vi "Get Compatible Interfaces.vi"(8 "error in (no error)":errorcluster, 10 "Interface Filter":T1[](array[typedef]), 11 "fpga resources":T3[](array[typedef]) {"fpga cd" format="%.0x"}) -> (0 "error out":errorcluster, 2 "Compatible Interface Names":string[](array[string]), 3 "fpga resources out":T3[](array[typedef]) {"fpga cd" format="%.0x"})   [LabVIEW 2016, in "FPGA RM System Definition API.lvlib"]
uses:
  FPGA RM System Definition API.lvlib
  Types/resources.ctl
  <vilib>/NI Veristand/Custom Device API/Custom Device Item Ref.ctl
  Types/fpga resource.ctl
  Types/Channel Type.ctl
  Shared/Requested Resource.ctl
  Shared/FPGA RM Shared API.lvlib
  <vilib>/NI VeriStand/Custom Device API/Custom Device API.lvlib
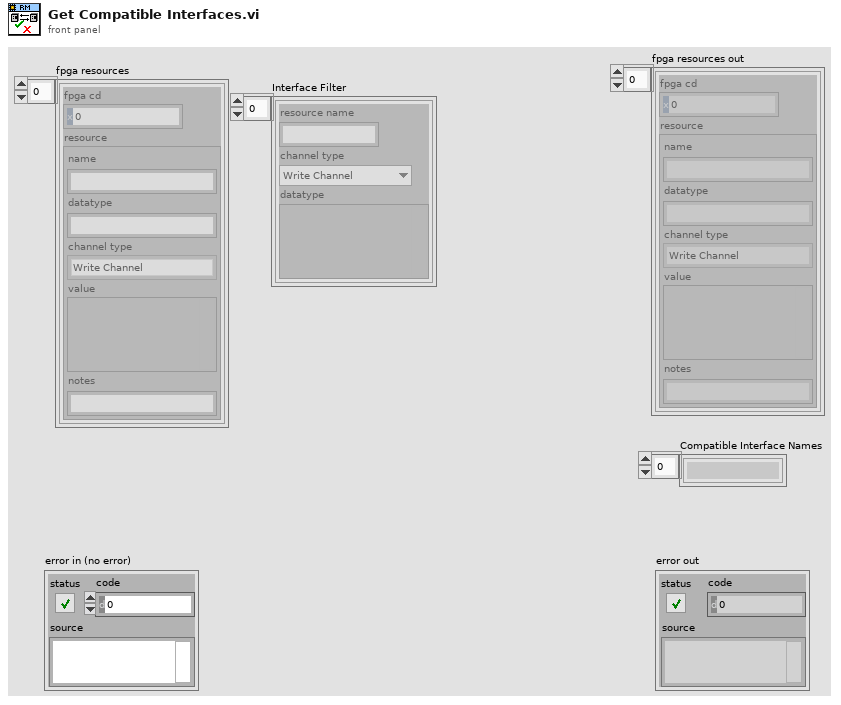
[diagram p1: front panel]
types:
  T1 = typedef "FPGA RM Shared API.lvlib/Requested Resource.ctl" = cluster{"resource name":string, "channel type":T2, "datatype":variant}
  T2 = typedef "FPGA RM Shared API.lvlib/Channel Type.ctl" = enum16{"Write Channel", "Read Channel", "Write Waveform", "Read Waveform"}
  T3 = typedef "FPGA RM System Definition API.lvlib/resources.ctl" = cluster{"fpga cd":T4, "resource":T5}
  T4 = typedef "Custom Device API.lvlib/Custom Device Item Ref.ctl" = u64
  T5 = typedef "FPGA RM Shared API.lvlib/fpga resource.ctl" = cluster{"name":string, "datatype":string, "channel type":T2, "value":variant, "notes":string}
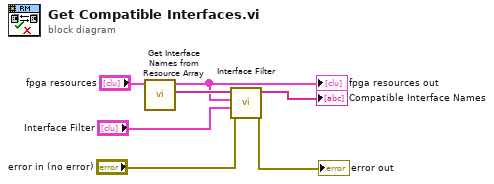
[diagram p0: block diagram]
diagram:
  n1 = call "Get Interface Names from Resource Array.vi"("fpga resources"="fpga resources") -> ("Interface Names"=w6:string[], "fpga resources out"=w4:T3[])  [unwired: 9 in]
  "fpga resources out" <- w4
  n2 = call "Interface Filter.vi"("error in (no error)"="error in (no error)", "Interface Filter"="Interface Filter", "fpga resources"=w4, "Interface Names"=w6) -> ("error out"=→"error out":errorcluster, "Compatible Interface Names"=→"Compatible Interface Names":string[])  [unwired: 6 in]
